vi "Custom Error_ Check FIFO Time Out.vi"(8 "error in":errorcluster, 11 "FPGA VI Reference In":refnum<k20>) -> (0 "error out":errorcluster, 3 "FPGA VI Reference Out":refnum<k20>)   [LabVIEW 2012]
uses:
  <vilib>/rvi/errors/niLvFpgaAdjustHostInterfaceError.vi
  <vilib>/rvi/interface/nirviReadWriteControl/nirviReadWriteControl.xnode
  NiFpgaLv.dll
  <vilib>/rvi/interface/Simulation/niFpgaSimulationCallBeginRW.vi
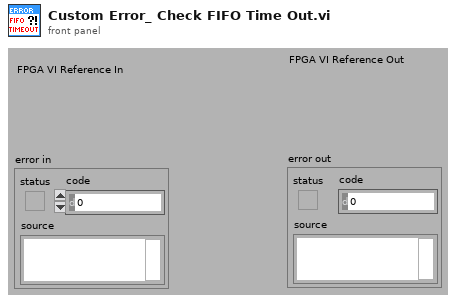
[diagram p1: front panel]
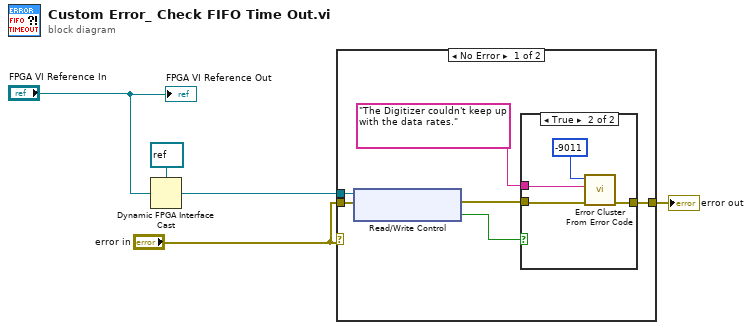
[diagram p0: block diagram]
diagram:
  n1 = Dynamic FPGA Interface Cast(Session In=refnum<k20> refnum ("Type"), Type="FPGA VI Reference In") -> (Session Out=w2:refnum<k20>)
  n2 = case shown="No Error" "error in" {
    tunnel: w2 -> [w11 _]
    tunnel: "error in" -> [w10 w17]
    tunnel: [w7 w17] -> w1
    frame No Error {
      n3 = xnode "Read/Write Control"("FPGA VI Reference In"=w11, "error in"=w10) -> ("error out"=w8:errorcluster, "FIFO Timed Out?"=w9:bool)  [unwired: 1 out]
      n4 = case shown="True" w9 {
        tunnel: w8 -> [w12 w14]
        tunnel: [w12 w16] -> w7
        tunnel: "The Digitizer couldn't keep up with the data rates." ("source") -> [_ w13]
        frame False {
        }
        frame True {
          n5 = call <vilib>:"Error Cluster From Error Code.vi"("error in (no error)"=w14, "error message (\"\")"=w13, "error code (0)"=-9011 ("code")) -> ("error out"=w16:errorcluster)  [unwired: 6 in]
        }
      }
    }
    frame Error {
    }
  }
  "error out" <- w1
  "FPGA VI Reference Out" <- "FPGA VI Reference In"
